vi "CRYTotal Noise Calculator.vi"(0 "Input Signal":dbl[](array[numeric]) format="%.19f", 2 "window":u16, 5 "Fs":dbl, 11 "Type(Harm,Inter,Diff)":u16, 12 "Freq Array":dbl[](array[numeric])) -> (4 "Total Noise":dbl format="%.23f", 6 "Standard Error":dbl[](array[numeric]))   [LabVIEW 2013]
uses:
  <vilib>/Analysis/baseanly.llb/Mean (DBL).vi
  <vilib>/Analysis/2dsp.llb/Real FFT.vi
  <vilib>/Analysis/0measdsp.llb/Scaled Time Domain Window (DBL).vi
  <vilib>/Analysis/NI_AALPro.lvlib
  <vilib>/Analysis/NI_AALBase.lvlib
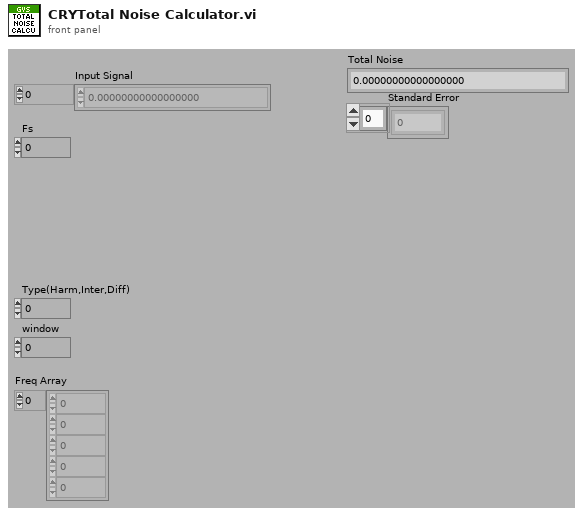
[diagram p1: front panel]
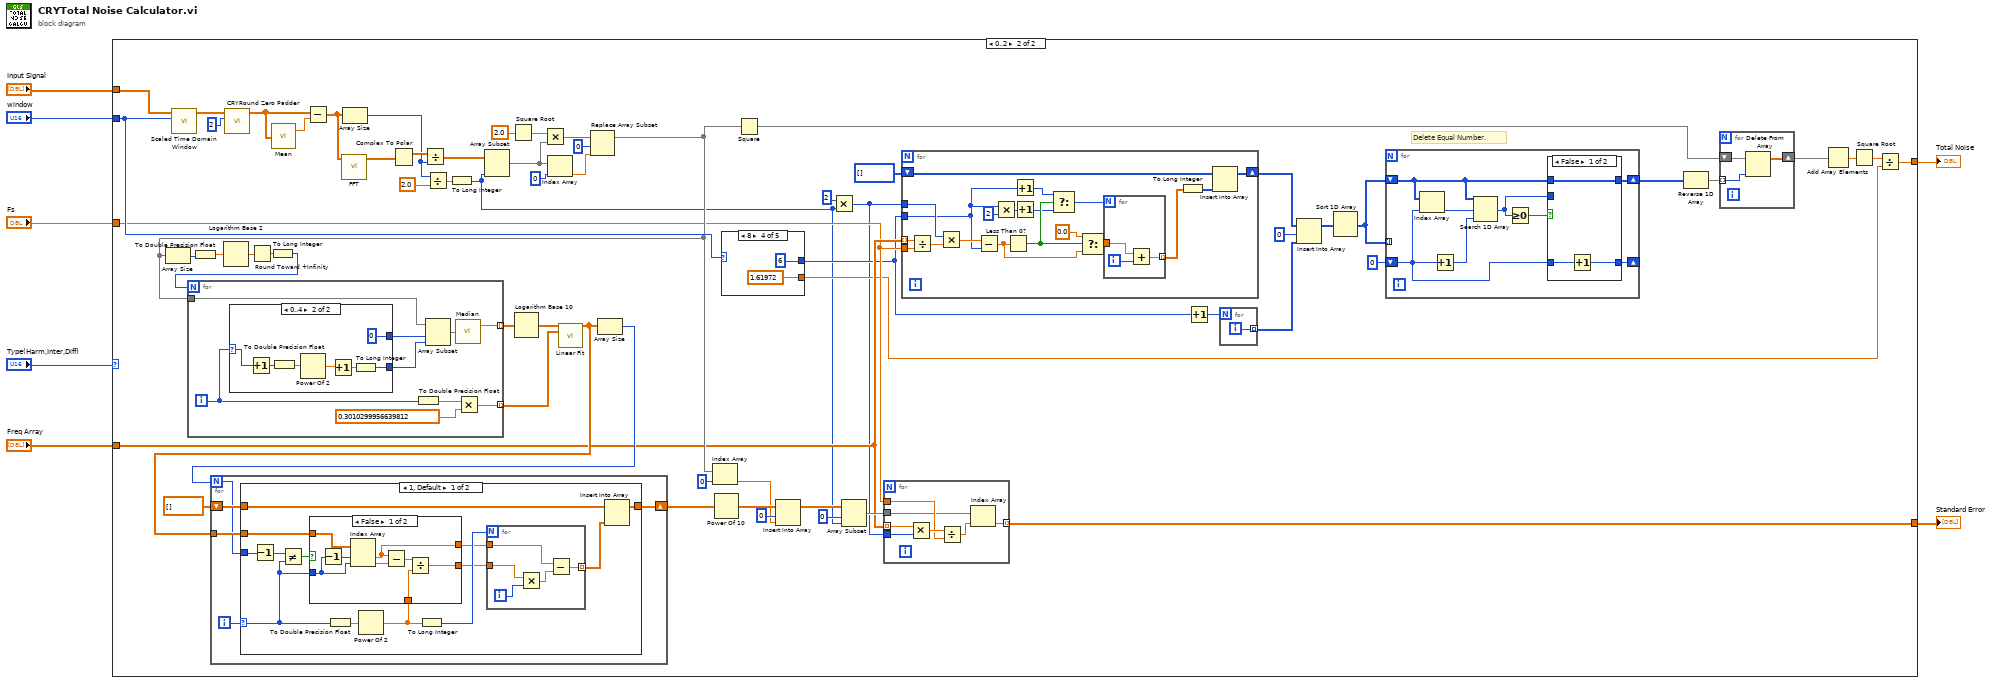
[diagram p0: block diagram]
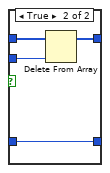
[diagram p3: hidden frame]
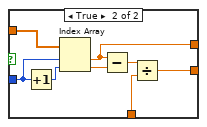
[diagram p4: hidden frame]
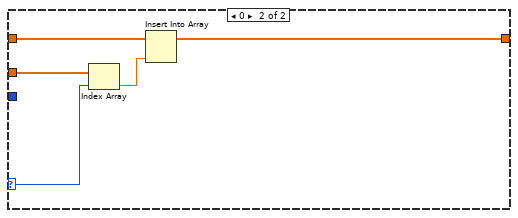
[diagram p5: hidden frame]
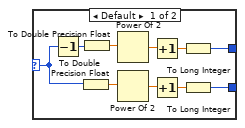
[diagram p6: hidden frame]
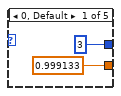
[diagram p7: hidden frame]
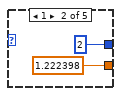
[diagram p8: hidden frame]
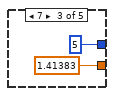
[diagram p9: hidden frame]
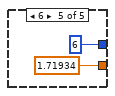
[diagram p10: hidden frame]
diagram:
  n1 = case shown="0..2" "Type(Harm,Inter,Diff)" {
    tunnel: "Fs" -> [_ w14]
    tunnel: "Input Signal" -> [_ w54]
    tunnel: [_ w30] -> w5
    tunnel: "Freq Array" -> [_ w15]
    tunnel: "window" -> [_ w52]
    tunnel: [_ w12] -> w2
    frame Default {
    }
    frame 0..2 {
      # "Delete Equal Number."
      n2 = call-poly <vilib>:"Scaled Time Domain Window.vi"("window"=w52, "X"=w54) -> ("Windowed X"=w60:dbl[])  [unwired: 7 in, 2 out]
      n3 = call "CRYRound Zero Padder.vi"("Significant Digit"=u8 2, "Vector in"=w60) -> ("Zero Padder Vector out"=w58:dbl[])  [unwired: 8 in, 1 out]
      n4 = call-poly <vilib>:"Mean.vi"("X"=w58) -> ("mean"=w57:dbl)  [unwired: 1 out]
      n5 = Subtract(x=w58, y=w57) -> (x-y=w53:dbl[])
      n6 = call-poly <vilib>:"FFT.vi"("X"=w53) -> ("FFT {X}"=w63:cdb[])  [unwired: 9 in, 1 out]
      n7 = Array Size(array=w53) -> (size(s)=w61:i32)
      n8 = Complex To Polar(r * e^(i*theta)=w63) -> (r=w64:dbl[])  [unwired: 1 out]
      n9 = Divide(x=w64, y=w61) -> (x/y=w62:dbl[])
      n10 = Divide(x=w61, y=2.0) -> (x/y=w66:dbl)
      n11 = To Long Integer(number=w66) -> (32bit integer=w9:i32)
      n12 = Array Subset(array=w62, length=w9) -> (w68:dbl[])  [unwired: 1 in]
      n13 = Square Root(x=2.0 ("y")) -> (sqrt(x)=w55:dbl)
      n14 = Multiply(x=w55, y=w68) -> (x*y=w51:dbl[])
      n15 = Index Array(array=w68, index=0) -> (element=w70:dbl)
      n16 = Replace Array Subset(array=w51, new element=w70, index=0) -> (w34:dbl[])
      n17 = Array Size(array=w34) -> (size(s)=w50:i32)
      n18 = To Double Precision Float(number=w50) -> (double precision float=w48:dbl)
      n19 = Logarithm Base 2(1:w48) -> (0:w49:dbl)
      n20 = Round Toward +Infinity(x=w49) -> (ceil(x): smallest int >= x=w47:dbl)
      n21 = To Long Integer(number=w47) -> (32bit integer=w44:i32)
      n22 = for {
        N: w44 -> [_]
        tunnel: w34 -> [w169]
        tunnel: [w167] -> w46 mode=indexing
        tunnel: [w163] -> w45 mode=indexing
        i -> [w166]
        n23 = case shown="0..4" w166 {
          selector: w166 -> [w173 w187]
          tunnel: [w177 0 ("index")] -> w170
          tunnel: [w172 w182] -> w171
          frame Default {
            n24 = Decrement(x=w173) -> (x-1=w181:i32)
            n25 = To Double Precision Float(number=w173) -> (double precision float=w174:dbl)
            n26 = To Double Precision Float(number=w181) -> (double precision float=w180:dbl)
            n27 = Power Of 2(x=w180) -> (2^x=w179:dbl)
            n28 = Power Of 2(x=w174) -> (2^x=w175:dbl)
            n29 = Increment(x=w179) -> (x+1=w178:dbl)
            n30 = Increment(x=w175) -> (x+1=w176:dbl)
            n31 = To Long Integer(number=w178) -> (32bit integer=w177:i32)
            n32 = To Long Integer(number=w176) -> (32bit integer=w172:i32)
          }
          frame 0..4 {
            n33 = Increment(x=w187) -> (x+1=w186:i32)
            n34 = To Double Precision Float(number=w186) -> (double precision float=w185:dbl)
            n35 = Power Of 2(x=w185) -> (2^x=w184:dbl)
            n36 = Increment(x=w184) -> (x+1=w183:dbl)
            n37 = To Long Integer(number=w183) -> (32bit integer=w182:i32)
          }
        }
        n38 = To Double Precision Float(number=w166) -> (double precision float=w165:dbl)
        n39 = Array Subset(array=w169, index=w170, length=w171) -> (w168:dbl[])
        n40 = call <vilib>:"Median.vi"("X"=w168) -> ("median"=w167:dbl)  [unwired: 1 out]
        n41 = Multiply(x=w165, y=0.3010299956639812) -> (x*y=w163:dbl)
      }
      n42 = Logarithm Base 10(1:w46) -> (0:w43:dbl[])
      n43 = call <vilib>:"Linear Fit.vi"("Y"=w43, "X"=w45) -> ("Best Linear Fit"=w41:dbl[])  [unwired: 9 in, 4 out]
      n44 = Array Size(array=w41) -> (size(s)=w42:i32)
      n45 = for {
        N: w42 -> [w119]
        tunnel: w41 -> [w120]
        shift-right: [w121] -> w39
        shift-left: dbl[] [] -> [w122]
        i -> [w123]
        n46 = case shown="1, Default" w123 {
          selector: w123 -> [w133 w159]
          tunnel: w122 -> [w126 w162]
          tunnel: [w124 w161] -> w121
          tunnel: w120 -> [w131 w160]
          tunnel: w119 -> [w136 _]
          frame 1, Default {
            n47 = Decrement(x=w136) -> (x-1=w135:i32)
            n48 = Not Equal?(x=w135, y=w133) -> (x != y?=w134:bool)
            n49 = To Double Precision Float(number=w133) -> (double precision float=w132:dbl)
            n50 = Power Of 2(x=w132) -> (2^x=w130:dbl)
            n51 = case shown="False" w134 {
              tunnel: w133 -> [w143 w157]
              tunnel: w131 -> [w147 w155]
              tunnel: w130 -> [w146 w152]
              tunnel: [w144 w151] -> w127
              tunnel: [w145 w150] -> w128
              frame False {
                n52 = Decrement(x=w143) -> (x-1=w142:i32)
                n53 = Index Array(array=w147, index #1=w142, index #2=w143) -> (element #1=w145:dbl, element #2=w149:dbl)
                n54 = Subtract(x=w145, y=w149) -> (x-y=w148:dbl)
                n55 = Divide(x=w148, y=w146) -> (x/y=w144:dbl)
              }
              frame True {
                n56 = Increment(x=w157) -> (x+1=w156:i32)
                n57 = Index Array(array=w155, index #1=w157, index #2=w156) -> (element #1=w150:dbl, element #2=w154:dbl)
                n58 = Subtract(x=w150, y=w154) -> (x-y=w153:dbl)
                n59 = Divide(x=w153, y=w152) -> (x/y=w151:dbl)
              }
            }
            n60 = To Long Integer(number=w130) -> (32bit integer=w129:i32)
            n61 = for {
              N: w129 -> [_]
              tunnel: w128 -> [w138]
              tunnel: w127 -> [w140]
              tunnel: [w137] -> w125 mode=indexing
              i -> [w141]
              n62 = Multiply(x=w140, y=w141) -> (x*y=w139:dbl)
              n63 = Subtract(x=w138, y=w139) -> (x-y=w137:dbl)
            }
            n64 = Insert Into Array(array=w126, new element=w125) -> (w124:dbl[])  [unwired: 1 in]
          }
          frame 0 {
            n65 = Index Array(array=w160, index=w159) -> (element=w158:dbl)
            n66 = Insert Into Array(array=w162, new element=w158) -> (w161:dbl[])  [unwired: 1 in]
          }
        }
      }
      n67 = Index Array(array=w34, index=0) -> (element=w35:dbl)
      n68 = Power Of 10(x=w39) -> (10^x=w37:dbl[])
      n69 = case shown="8" w52 {
        tunnel: [3 ("length") 2 ("length") 5 ("length") 6 ("length") 6 ("length")] -> w13
        tunnel: [0.999133 ("y") 1.222398 ("y") 1.41383 ("y") 1.61972 ("y") 1.71934 ("y")] -> w10
        frame 0, Default {
        }
        frame 1 {
        }
        frame 7 {
        }
        frame 8 {
        }
        frame 6 {
        }
      }
      n70 = Square(x=w34) -> (x^2=w19:dbl[])
      n71 = Insert Into Array(array=w37, index=0, new element=w35) -> (w33:dbl[])
      n72 = Multiply(x=2 ("y"), y=w9) -> (x*y=w8:i32)
      n73 = Array Subset(array=w33, index=0, length=w9) -> (w31:dbl[])
      n74 = for {
        tunnel: w15 -> [w118] mode=indexing
        tunnel: w31 -> [w113]
        tunnel: w14 -> [w115]
        tunnel: w8 -> [w117]
        tunnel: [w112] -> w30 mode=indexing
        n75 = Multiply(x=w118, y=w117) -> (x*y=w116:dbl)
        n76 = Divide(x=w116, y=w115) -> (x/y=w114:dbl)
        n77 = Index Array(array=w113, index=w114) -> (element=w112:dbl)
      }
      n78 = for {
        tunnel: w14 -> [w108]
        tunnel: w8 -> [w106]
        tunnel: w15 -> [w105] mode=indexing
        tunnel: w13 -> [w94]
        shift-right: [w92] -> w25
        shift-left: i32[] [] ("Ft") -> [w93]
        n79 = Divide(x=w105, y=w108) -> (x/y=w107:dbl)
        n80 = Multiply(x=w106, y=w107) -> (x*y=w104:dbl)
        n81 = Subtract(x=w104, y=w94) -> (x-y=w103:dbl)
        n82 = Multiply(x=w94, y=2) -> (x*y=w99:i32)
        n83 = Less Than 0?(x=w103) -> (x < 0?=w98:bool)
        n84 = Increment(x=w94) -> (x+1=w97:i32)
        n85 = Increment(x=w99) -> (x+1=w96:i32)
        n86 = Select(t=w97, s=w98, f=w96) -> (s? t:f=w95:i32)
        n87 = Select(t=0.0, s=w98, f=w103) -> (s? t:f=w101:dbl)
        n88 = for {
          N: w95 -> [_]
          tunnel: w101 -> [w111]
          tunnel: [w109] -> w91 mode=indexing
          i -> [w110]
          n89 = Add(x=w111, y=w110) -> (x+y=w109:dbl)
        }
        n90 = To Long Integer(number=w91) -> (32bit integer=w90:i32[])
        n91 = Insert Into Array(array=w93, new element=w90) -> (w92:i32[])  [unwired: 1 in]
      }
      n92 = Increment(x=w13) -> (x+1=w28:i32)
      n93 = for {
        N: w28 -> [_]
        tunnel: [w89] -> w27 mode=indexing
        i -> [w89]
      }
      n94 = Insert Into Array(array=w25, index=0 ("index (row)"), new element=w27) -> (w24:i32[])
      n95 = Sort 1D Array(array=w24) -> (sorted array=w22:i32[])
      n96 = for {
        shift-right: [w74] -> w21
        shift-left: w22 -> [w81]
        shift-right: [w75] -> _
        shift-left: 0 ("index (row)") -> [w76]
        tunnel: w22 -> [_] mode=indexing
        n97 = Index Array(array=w81, index=w76) -> (element=w80:i32)
        n98 = Increment(x=w76) -> (x+1=w79:i32)
        n99 = Search 1D Array(1D array=w81, element=w80, start index (0)=w79) -> (index of element=w77:i32)
        n100 = Greater Or Equal To 0?(x=w77) -> (x >= 0?=w78:bool)
        n101 = case shown="False" w78 {
          tunnel: w81 -> [w84 w88]
          tunnel: [w84 w87] -> w74
          tunnel: w77 -> [_ w86]
          tunnel: w76 -> [w83 w85]
          tunnel: [w82 w85] -> w75
          frame False {
            n102 = Increment(x=w83) -> (x+1=w82:i32)
          }
          frame True {
            n103 = Delete From Array(array=w88, index=w86) -> (array with subset deleted=w87:i32[])  [unwired: 1 in, 1 out]
          }
        }
      }
      n104 = Reverse 1D Array(array=w21) -> (reversed array=w20:i32[])
      n105 = for {
        tunnel: w20 -> [w72] mode=indexing
        shift-right: [w71] -> w16
        shift-left: w19 -> [w73]
        n106 = Delete From Array(array=w73, index=w72) -> (array with subset deleted=w71:dbl[])  [unwired: 1 in, 1 out]
      }
      n107 = Add Array Elements(numeric array=w16) -> (sum=w18:dbl)
      n108 = Square Root(x=w18) -> (sqrt(x)=w17:dbl)
      n109 = Divide(x=w17, y=w10) -> (x/y=w12:dbl)
    }
  }
  "Total Noise" <- w2
  "Standard Error" <- w5
